vi "Facade.vi"(0 "Data In":T8, 2 "Display State In":T2, 3 "Container State":T7) -> (6 "Data Out":T8, 7 "Display State Out":T2, 8 "Action":T1)   [LabVIEW 2020, in "KTable.xctl"]
uses:
  KTable.xctl
  Data.ctl
  <vilib>/_xctls/Container State.ctl
  State.ctl
  ColumnSpec.ctl
  ColumnType.ctl
  Table Properties.ctl
  Events.ctl
  Event Data.ctl
  Event Type.ctl
  <vilib>/_xctls/Action.ctl
  <vilib>/Utility/miscctls.llb/LVPositionTypeDef.ctl
  <vilib>/_xctls/XControlSupport.lvlib
panel:
  in  "Color":u32(colorbox)
  out "layout":bool
  in  "Ring":u16(ring)
  in  "Listbox":i32(listbox)
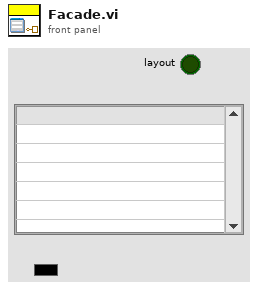
[diagram p1: front panel]
types:
  T1 = typedef "XControlSupport.lvlib/Action.ctl" = cluster{"Data Changed?":bool, "State Changed?":bool, "Action Name":string}
  T2 = typedef "KTable.xctl/State.ctl" = cluster{"Columns":T3[], "Listbox":refnum<vi>, "Default row":string[], "Properties":T5, "Events":T6, "Locked":bool[][], "Size":cluster{"Rows":i32, "Columns":i32}, "rings":i32[][], "DefColors":u32[], "highlight row":bool}
  T3 = typedef "KTable.xctl/ColumnSpec.ctl" = cluster{"Name":string, "Type":T4, "Width":i32, "Strings":string[], "Position":enum16{"Left", "Center", "Right"}, "locked":bool, "cds":cluster{"Strings":string[]}[][], "Hide NaN":bool}
  T4 = typedef "KTable.xctl/ColumnType.ctl" = enum16{"String", "Enum", "Int", "Double", "Boolean", "Ring", "Formula", "Color"}
  T5 = typedef "KTable.xctl/Table Properties.ctl" = cluster{"Vertical scrollbar":bool, "User add/delete":bool, "Max rows":i32, "Row headers":bool}
  T6 = typedef "KTable.xctl/Events.ctl" = cluster{"Items Changed":refnum<user-event>}
  T7 = typedef "XControlSupport.lvlib/Container State.ctl" = cluster{"Indicator?":bool, "Run Mode?":bool, " Refnum":refnum<vi>}
  T8 = typedef "KTable.xctl/Data.ctl" = u16
  T9 = typedef "KTable.xctl/Event Data.ctl" = cluster{"Type":T10, "New row":i32, "Old row":i32, "Data":variant}
  T10 = typedef "KTable.xctl/Event Type.ctl" = enum16{"None", "Selection", "Edit", "Insert", "Delete", "Up", "Down", "Duplicate"}
  T11 = typedef "LVPositionTypeDef.ctl" = cluster{"Left":i32, "Top":i32}
  T12 = typedef "LVRectTypeDef.ctl" = cluster{"Left":i16, "Top":i16, "Right":i16, "Bottom":i16}
  T13 = typedef "LVPoint32TypeDef.ctl" = cluster{"Horizontal":i32, "Vertical":i32}
  T14 = typedef "LVRowAndColumnTypeDef.ctl" = cluster{"Row":i32, "Column":i32}
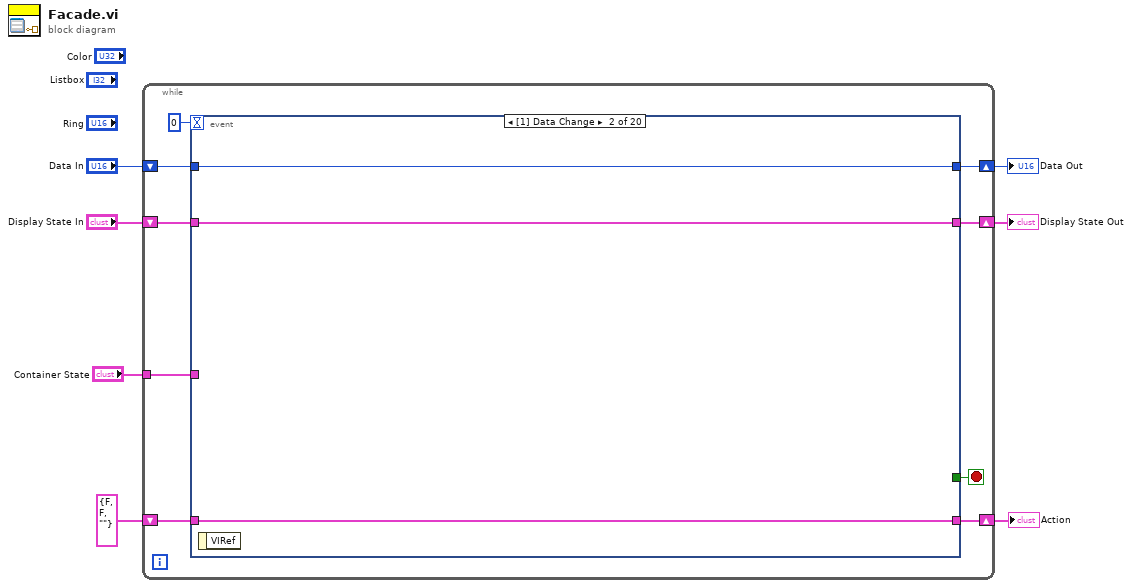
[diagram p0: block diagram]
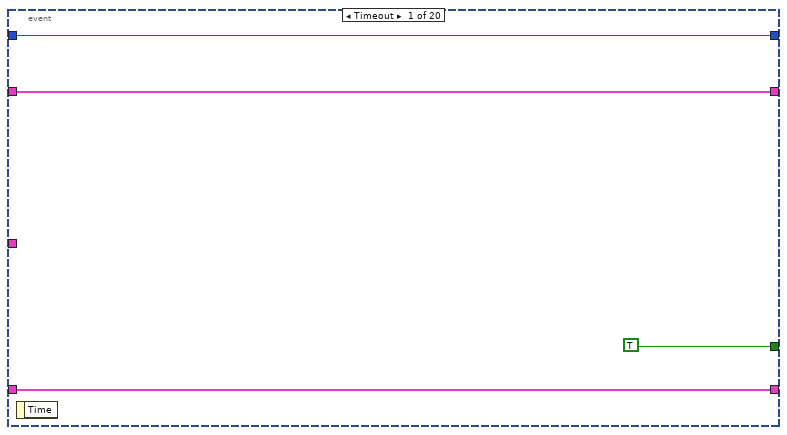
[diagram p2: hidden frame]
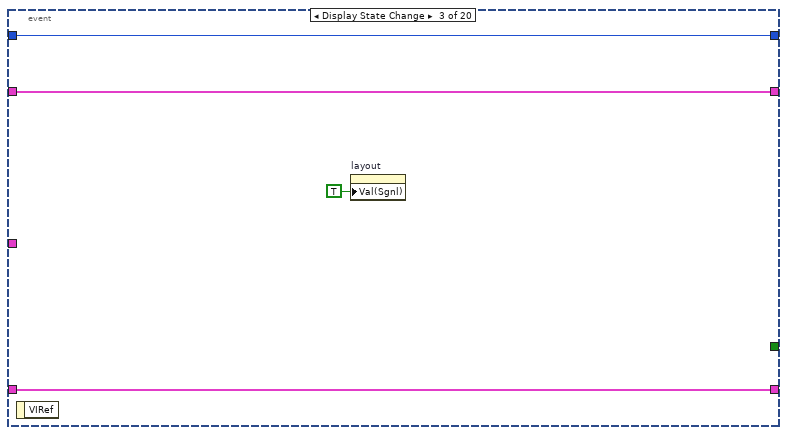
[diagram p3: hidden frame]
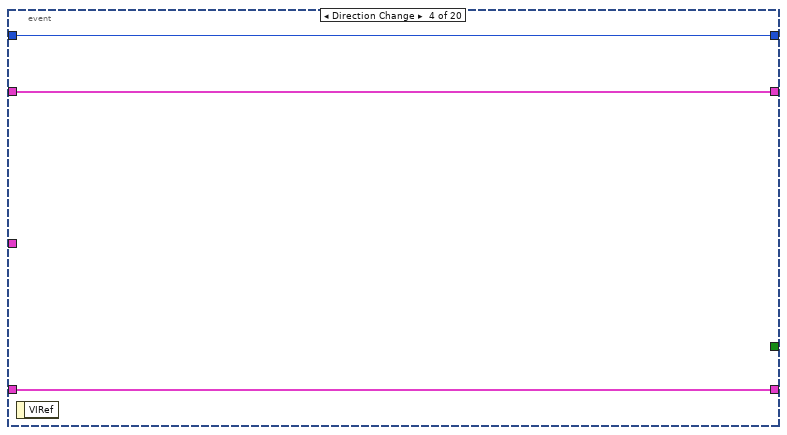
[diagram p4: hidden frame]
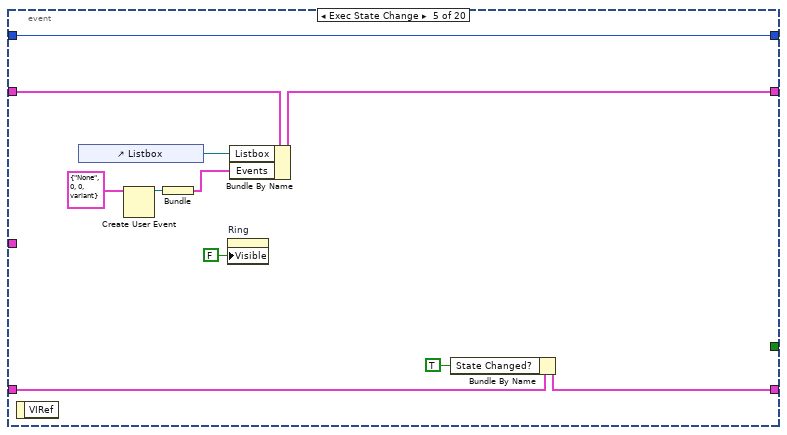
[diagram p5: hidden frame]
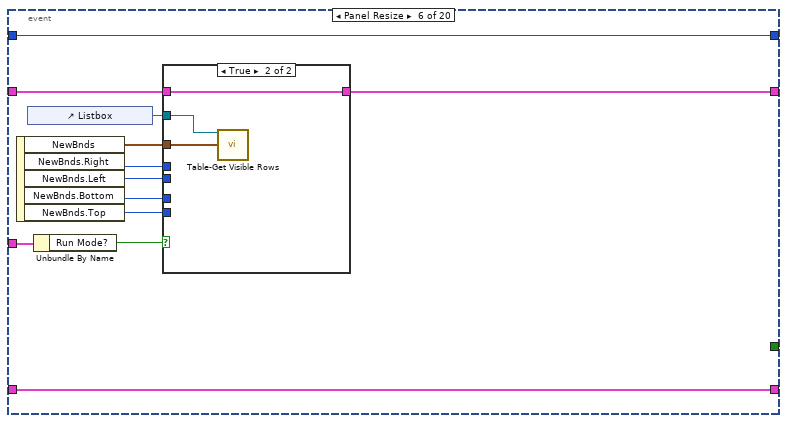
[diagram p6: hidden frame]
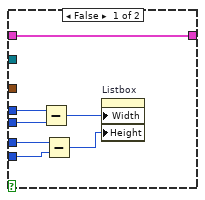
[diagram p7: hidden frame]
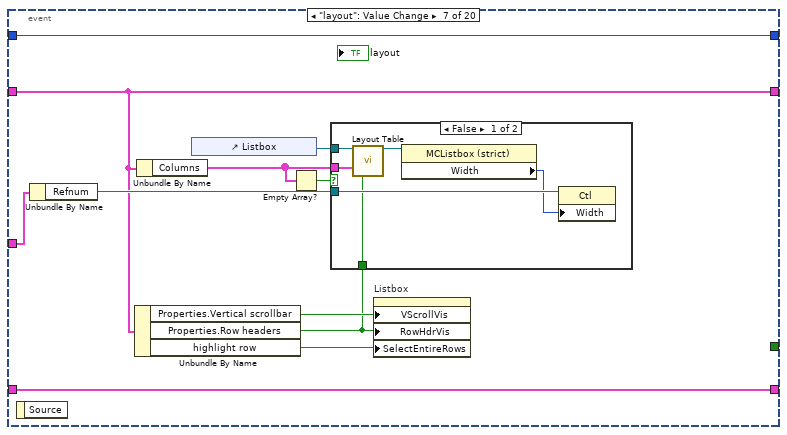
[diagram p8: hidden frame]
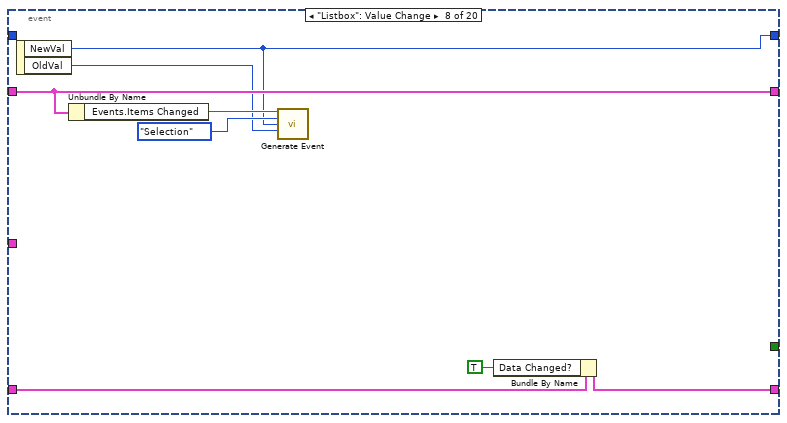
[diagram p10: hidden frame]
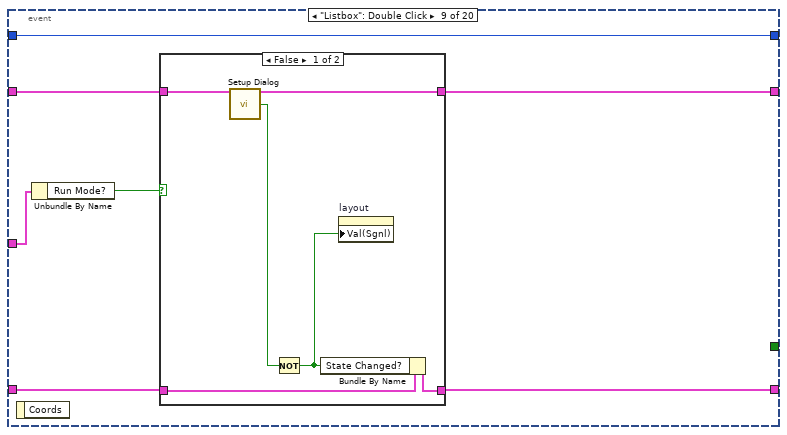
[diagram p11: hidden frame]
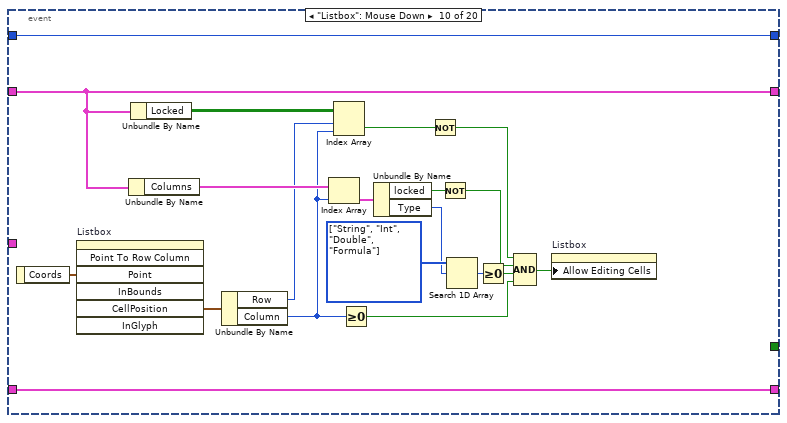
[diagram p13: hidden frame]
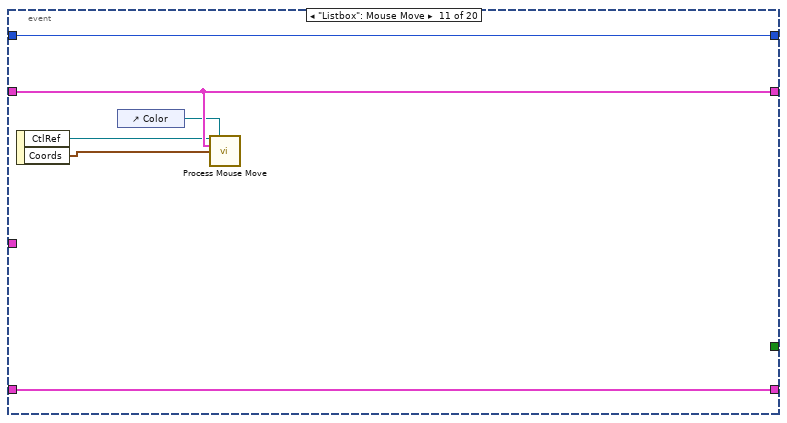
[diagram p14: hidden frame]
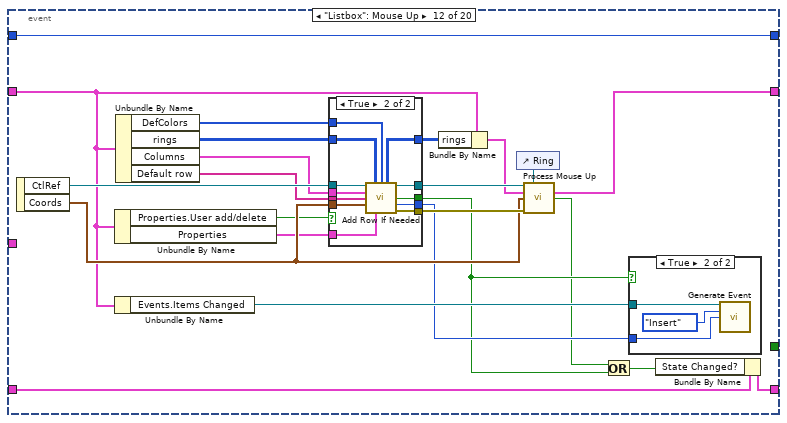
[diagram p15: hidden frame]
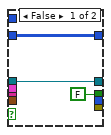
[diagram p16: hidden frame]
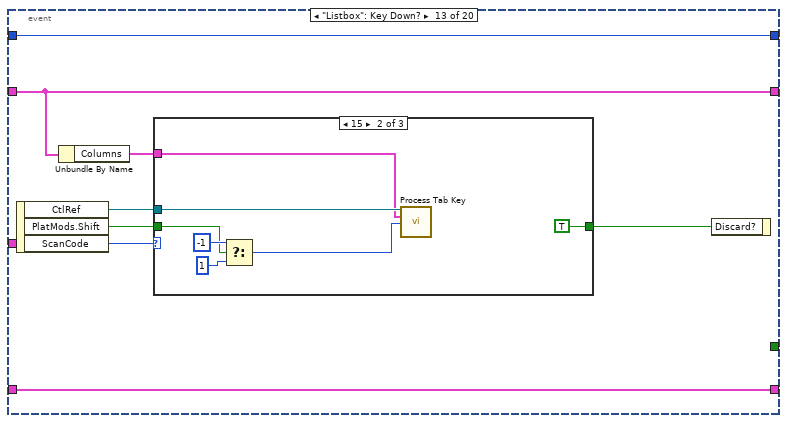
[diagram p18: hidden frame]
diagram:
  n1 = while {
    shift-right: [w15] -> w4
    shift-left: "Display State In" -> [w16]
    tunnel: "Container State" -> [w12]
    shift-right: [w10] -> w7
    shift-left: "Data In" -> [w11]
    shift-right: [w8] -> w2
    shift-left: T1 {"Data Changed?"=FALSE, "State Changed?"=FALSE, "Action Name"=""} ("Action") -> [w9]
    stop <- w14 stop-if-true
    n2 = event shown="[1] Data Change" {
      selector: _ -> [_ _ _ _ _ _ _ _ _ _ _ _ _ _ _ _ _ _ _ _]
      dyn-events: _ -> [_ _ _ _ _ _ _ _ _ _ _ _ _ _ _ _ _ _ _ _]
      timeout: 0 -> [_ _ _ _ _ _ _ _ _ _ _ _ _ _ _ _ _ _ _ _]
      tunnel: w16 -> [w18 w22 w27 w30 w41 w45 w65 w85 w93 w109 w127 w140 w173 w195 w208 w216 w230 w251 w272 w288]
      tunnel: [w18 w22 w27 w30 w38 w44 w65 w85 w89 w109 w127 w131 w173 w195 w208 w216 w230 w245 w272 w288] -> w15
      tunnel: [TRUE _ _ _ _ _ _ _ _ _ _ _ _ _ _ _ _ _ _ _] -> w14
      tunnel: w12 -> [_ _ _ _ _ w47 w71 _ w94 _ _ _ _ _ _ _ _ _ _ _]
      tunnel: w11 -> [w17 w23 w26 w29 w40 w53 w74 _ w95 w123 w129 w152 w178 w202 w212 w218 w236 w264 w284 w287]
      tunnel: [w17 w23 w26 w29 w40 w53 w74 w82 w95 w123 w129 w152 w178 w202 w212 w218 w236 w264 w284 w287] -> w10
      tunnel: [w19 w21 w25 w28 w36 w52 w73 w87 w90 w122 w128 w135 w177 w197 w211 w217 w232 w253 w274 w286] -> w8
      tunnel: w9 -> [w19 w21 w25 w28 w39 w52 w73 w88 w92 w122 w128 w151 w177 w201 w211 w217 w235 w263 w283 w286]
      event Timeout {
        n3 = event-data() -> ()  [unwired: 1 in, 1 out]
      }
      event Data Change {
        n4 = event-data() -> ()  [unwired: 1 in, 1 out]
      }
      event Display State Change {
        n5 = event-data() -> ()  [unwired: 1 in, 1 out]
        n6 = property on="layout" class="Bool (strict)"("Val(Sgnl)"=TRUE ("Value (Signaling)")) -> ()  [unwired: 2 in, 2 out]
      }
      event Direction Change {
        n7 = event-data() -> ()  [unwired: 1 in, 1 out]
      }
      event Exec State Change {
        n8 = event-data() -> ()  [unwired: 1 in, 1 out]
        n9 = control-ref of="Listbox"() -> (w37:refnum<vi>)
        n10 = Create User Event(user event datatype=T9 {"Type"=enum."None", "New row"=0, "Old row"=0, "Data"=variant} ("Event Data")) -> (user event=w33:refnum<user-event>)  [unwired: 1 in, 1 out]
        n11 = Bundle("Event Data"=w33) -> (w31:cluster{"Event Data":refnum<user-event>})  [unwired: 1 in]
        n12 = property on="Ring" class="Ring (strict)"("Visible"=FALSE) -> ()  [unwired: 2 in, 2 out]
        n13 = Bundle By Name(cluster=w41, "Listbox"=w37, "Events"=w31) -> (w38:T2)
        n14 = Bundle By Name(cluster=w39, "State Changed?"=TRUE) -> (w36:T1)
      }
      event Panel Resize {
        n15 = event-data() -> ("NewBnds"=w46:T12, "NewBnds.Right"=w50:i16, "NewBnds.Left"=w51:i16, "NewBnds.Bottom"=w48:i16, "NewBnds.Top"=w49:i16)  [unwired: 1 in]
        n16 = control-ref of="Listbox"() -> (w42:refnum<vi>)
        n17 = Unbundle By Name(w47) -> ("Run Mode?"=w43:bool)
        n18 = case shown="True" w43 {
          tunnel: w51 -> [w60 _]
          tunnel: w50 -> [w59 _]
          tunnel: w49 -> [w58 _]
          tunnel: w48 -> [w57 _]
          tunnel: w46 -> [_ w63]
          tunnel: w45 -> [w54 w61]
          tunnel: [w54 w61] -> w44
          tunnel: w42 -> [_ w62]
          frame False {
            n19 = Subtract(x=w59, y=w60) -> (x-y=w56:i16)
            n20 = Subtract(x=w57, y=w58) -> (x-y=w55:i16)
            n21 = property on="Listbox" class="MCListbox (strict)"("Width"=w56, "Height"=w55) -> ()  [unwired: 2 in, 2 out]
          }
          frame True {
            n22 = call "Table-Get Visible Rows.vi"("reference"=w62, "Bounds"=w63) -> ()  [unwired: 13 in, 1 out]
          }
        }
      }
      event "layout": Value Change {
        n23 = event-data() -> ()  [unwired: 1 in, 1 out]
        n24 = Unbundle By Name(w71) -> ("Refnum"=w70:refnum<vi>)
        n25 = Unbundle By Name(w65) -> ("Properties.Vertical scrollbar"=w67:bool, "Properties.Row headers"=w66:bool, "highlight row"=w64:bool)
        n26 = Unbundle By Name(w65) -> ("Columns"=w69:T3[])
        n27 = control-ref of="Listbox"() -> (w72:refnum<vi>)
        n28 = Empty Array?(array=w69) -> (empty?=w68:bool)
        n29 = case shown="False" w68 {
          tunnel: w72 -> [w80 _]
          tunnel: w70 -> [w78 _]
          tunnel: w69 -> [w76 _]
          tunnel: w66 -> [w75 _]
          frame False {
            n30 = call "Layout Table.vi"("Listbox Ref"=w80, "Columns"=w76, "row headers"=w75) -> ("reference out"=w79:refnum<vi>)  [unwired: 12 in]
            n31 = property class="MCListbox (strict)"(reference=w79) -> ("Width"=w77:u32)  [unwired: 1 in, 2 out]
            n32 = property class="Ctl"(reference=w78, "Width"=w77) -> ()  [unwired: 1 in, 2 out]
          }
          frame True {
          }
        }
        n33 = property on="Listbox" class="MCListbox (strict)"("VScrollVis"=w67, "RowHdrVis"=w66, "SelectEntireRows"=w64) -> ()  [unwired: 2 in, 2 out]
      }
      event "Listbox": Value Change {
        n34 = event-data() -> ("NewVal"=w82:i32, "OldVal"=w81:i32)  [unwired: 1 in]
        n35 = Unbundle By Name(w85) -> ("Events.Items Changed"=w84:refnum<user-event>)
        n36 = call "Generate Event.vi"("Event"=w84, "Type"=Event_Type."Selection", "New row"=w82, "Old row"=w81) -> ()  [unwired: 11 in, 1 out]
        n37 = Bundle By Name(cluster=w88, "Data Changed?"=TRUE) -> (w87:T1)
      }
      event "Listbox": Double Click {
        n38 = event-data() -> ()  [unwired: 1 in, 1 out]
        n39 = Unbundle By Name(w94) -> ("Run Mode?"=w91:bool)
        n40 = case shown="False" w91 {
          tunnel: w93 -> [w101 w102]
          tunnel: w92 -> [w99 w103]
          tunnel: [w98 w103] -> w90
          tunnel: [w100 w102] -> w89
          frame False {
            n41 = call "Setup Dialog.vi"("State In"=w101) -> ("State Out"=w100:T2, "canceled?"=w97:bool)  [unwired: 13 in]
            n42 = Not(x=w97) -> (.not. x?=w96:bool)
            n43 = Bundle By Name(cluster=w99, "State Changed?"=w96) -> (w98:T1)
            n44 = property on="layout" class="Bool (strict)"("Val(Sgnl)"=w96) -> ()  [unwired: 2 in, 2 out]
          }
          frame True {
          }
        }
      }
      event "Listbox": Mouse Down {
        w117 = T4[] [enum."String", enum."Int", enum."Double", enum."Formula"] items=["String", "Enum", "Int", "Double", "Boolean", "Ring", "Formula", "Color"] ("y")
        n45 = event-data() -> ("Coords"=w121:T13)  [unwired: 1 in]
        n46 = invoke on="Listbox" class="MCListbox (strict)" method="Point To Row Column"("Point"=w121) -> ("CellPosition"=w119:T14)  [unwired: 6 in, 6 out]
        n47 = Unbundle By Name(w109) -> ("Columns"=w120:T3[])
        n48 = Unbundle By Name(w109) -> ("Locked"=w113:bool[][])
        n49 = Unbundle By Name(w119) -> ("Row"=w112:i32, "Column"=w105:i32)
        n50 = Index Array(array=w120, index=w105) -> (element=w118:T3)
        n51 = Index Array(array=w113, index (row)=w112, index (col)=w105) -> (element=w110:bool)
        n52 = Greater Or Equal To 0?(x=w105) -> (x >= 0?=w104:bool)
        n53 = Unbundle By Name(w118) -> ("locked"=w107:bool, "Type"=w116:T4)
        n54 = Not(x=w110) -> (.not. x?=w108:bool)
        n55 = Not(x=w107) -> (.not. x?=w106:bool)
        n56 = Search 1D Array(1D array=w117, element=w116) -> (index of element=w115:i32)  [unwired: 1 in]
        n57 = Greater Or Equal To 0?(x=w115) -> (x >= 0?=w114:bool)
        n58 = Compound Arithmetic op=AND(w108, w106, w114, w104) -> (w111:bool)
        n59 = property on="Listbox" class="MCListbox (strict)"("Allow Editing Cells"=w111) -> ()  [unwired: 2 in, 2 out]
      }
      event "Listbox": Mouse Move {
        n60 = event-data() -> ("CtlRef"=w125:refnum<vi>, "Coords"=w124:T13)  [unwired: 1 in]
        n61 = control-ref of="Color"() -> (w126:refnum<vi>)
        n62 = call "Process Mouse Move.vi"("Listbox"=w125, "Color Box"=w126, "State in"=w127, "Coords"=w124) -> ()  [unwired: 10 in, 2 out]
      }
      event "Listbox": Mouse Up {
        n63 = event-data() -> ("CtlRef"=w149:refnum<vi>, "Coords"=w145:T13)  [unwired: 1 in]
        n64 = Unbundle By Name(w140) -> ("Properties.User add/delete"=w142:bool, "Properties"=w139:T5)
        n65 = Unbundle By Name(w140) -> ("Events.Items Changed"=w144:refnum<user-event>)
        n66 = Unbundle By Name(w140) -> ("DefColors"=w130:u32[], "rings"=w138:i32[][], "Columns"=w141:T3[], "Default row"=w147:string[])
        n67 = case shown="True" w142 {
          tunnel: w149 -> [w155 w167]
          tunnel: [w155 w166] -> w148
          tunnel: w147 -> [_ w165]
          tunnel: [_ w164] -> w146
          tunnel: w145 -> [_ w163]
          tunnel: w141 -> [_ w162]
          tunnel: [FALSE ("row added?") w161] -> w133
          tunnel: [_ w160] -> w143
          tunnel: w139 -> [_ w159]
          tunnel: w138 -> [w153 w158]
          tunnel: [w153 w157] -> w136
          tunnel: w130 -> [_ w156]
          frame False {
          }
          frame True {
            n68 = call "Add Row If Needed.vi"("Listbox In"=w167, "rings in"=w158, "DefColors"=w156, "Columns"=w162, "Default"=w165, "Coords"=w163, "Properties"=w159) -> ("rings out"=w157:i32[][], "Listbox out"=w166:refnum<vi>, "row added?"=w161:bool, "Row"=w160:i32, "error out"=w164:errorcluster)  [unwired: 4 in]
          }
        }
        n69 = Bundle By Name(cluster=w140, "rings"=w136) -> (w137:T2)
        n70 = control-ref of="Ring"() -> (w150:refnum<vi>)
        n71 = call "Process Mouse Up.vi"("Listbox"=w148, "Ring"=w150, "State in"=w137, "Coords"=w145, "error in (no error)"=w146) -> ("State out"=w131:T2, "state changed"=w132:bool)  [unwired: 8 in, 1 out]
        n72 = Or(x=w132, y=w133) -> (x .or. y?=w134:bool)
        n73 = case shown="True" w133 {
          tunnel: w144 -> [_ w170]
          tunnel: w143 -> [_ w168]
          frame False {
          }
          frame True {
            n74 = call "Generate Event.vi"("Event"=w170, "Type"=Event_Type."Insert", "New row"=w168) -> ()  [unwired: 12 in, 1 out]
          }
        }
        n75 = Bundle By Name(cluster=w151, "State Changed?"=w134) -> (w135:T1)
      }
      event "Listbox": Key Down? {
        n76 = event-data() -> ("CtlRef"=w171:refnum<vi>, "PlatMods.Shift"=w174:bool, "ScanCode"=w176:i16)  [unwired: 1 in]
        n77 = Unbundle By Name(w173) -> ("Columns"=w172:T3[])
        n78 = case shown="15" w176 {
          tunnel: [_ TRUE ("Shift") w186] -> w175
          tunnel: w174 -> [_ w183 w186]
          tunnel: w172 -> [_ w180 _]
          tunnel: w171 -> [_ w181 _]
          frame 0, Default {
          }
          frame 15 {
            n79 = Select(t=-1, s=w183, f=1) -> (s? t:f=w179:i32)
            n80 = call "Process Tab Key.vi"("MulticolumnListbox in"=w181, "Columns"=w180, "increment"=w179) -> ()  [unwired: 13 in]
          }
          frame 72, 80 {
          }
        }
        n81 = event-data("Discard?"=w175) -> ()  [unwired: 1 in, 1 out]
      }
      event "Listbox": Key Up {
        n82 = event-data() -> ("PlatMods.Shift"=w194:bool, "CtlRef"=w199:refnum<vi>, "ScanCode"=w200:i16)  [unwired: 1 in]
        n83 = local read "Listbox"() -> (w198:i32)
        n84 = Unbundle By Name(w195) -> ("Properties.User add/delete"=w193:bool)
        n85 = And(x=w193, y=w194) -> (x .and. y?=w187:bool)
        n86 = Unbundle By Name(w195) -> ("Events.Items Changed"=w192:refnum<user-event>)
        n87 = Unbundle By Name(w195) -> ("Properties"=w189:T5, "Columns"=w188:T3[])
        n88 = call "Process Keystroke.vi"("Listbox"=w199, "can move"=w187, "ScanCode"=w200, "Row"=w198, "Properties"=w189, "Columns"=w188) -> ("Event type"=w191:T10, "Row Out"=w190:i32, "data changed?"=w196:bool)  [unwired: 6 in, 1 out]
        n89 = case shown="True" w196 {
          tunnel: w192 -> [_ w206]
          tunnel: w191 -> [_ w205]
          tunnel: w190 -> [_ w204]
          tunnel: w198 -> [_ w203]
          frame False {
          }
          frame True {
            n90 = call "Generate Event.vi"("Event"=w206, "Type"=w205, "New row"=w204, "Old row"=w203) -> ()  [unwired: 11 in, 1 out]
          }
        }
        n91 = Bundle By Name(cluster=w201, "Data Changed?"=w196) -> (w197:T1)
      }
      event "Listbox": Edit Cell {
        n92 = event-data() -> ("Coords.Row"=w207:i32)  [unwired: 1 in]
        n93 = Unbundle By Name(w208) -> ("Events.Items Changed"=w210:refnum<user-event>)
        n94 = call "Generate Event.vi"("Event"=w210, "Type"=Event_Type."Edit", "New row"=w207) -> ()  [unwired: 12 in, 1 out]
      }
      event "Listbox": Shortcut Menu Activation? {
        n95 = event-data() -> ("MenuRef"=w215:refnum<k9>)  [unwired: 1 in]
        n96 = Unbundle By Name(w216) -> ("Properties.User add/delete"=w213:bool)
        n97 = Not(x=w213) -> (.not. x?=w214:bool)
        n98 = case shown="True" w213 {
          tunnel: w215 -> [_ w223]
          frame False {
          }
          frame True {
            n99 = Delete Menu Items(9:w223) -> (0:w222:errorcluster, 3:w221:refnum<k9>)  [unwired: 3 in]
            n100 = Insert Menu Items(6:w222, 7:string[] ["sc_delete_row", "sc_delete_all", "sc_duplicate_row"] ("item tags"), 8:string[] ["Delete selected row", "Delete all rows", "Duplicate selected row"] ("item names"), 9:w221) -> ()  [unwired: 2 in, 3 out]
          }
        }
        n101 = event-data("Discard?"=w214) -> ()  [unwired: 1 in, 1 out]
      }
      event "Listbox": Shortcut Menu Selection (User) {
        n102 = event-data() -> ("CtlRef"=w234:refnum<vi>, "ItemTag"=w225:string)  [unwired: 1 in]
        n103 = local read "Listbox"() -> (w233:i32)
        n104 = Unbundle By Name(w230) -> ("Events.Items Changed"=w229:refnum<user-event>)
        n105 = Unbundle By Name(w230) -> ("Properties"=w226:T5, "Columns"=w224:T3[])
        n106 = call "Process Menu.vi"("Listbox"=w234, "menu tag"=w225, "Row"=w233, "Properties"=w226, "Columns"=w224) -> ("Event type"=w228:T10, "Row Out"=w227:i32, "data changed?"=w231:bool)  [unwired: 7 in, 1 out]
        n107 = case shown="True" w231 {
          tunnel: w229 -> [_ w240]
          tunnel: w228 -> [_ w239]
          tunnel: w227 -> [_ w238]
          tunnel: w233 -> [_ w237]
          frame False {
          }
          frame True {
            n108 = call "Generate Event.vi"("Event"=w240, "Type"=w239, "New row"=w238, "Old row"=w237) -> ()  [unwired: 11 in, 1 out]
          }
        }
        n109 = Bundle By Name(cluster=w235, "Data Changed?"=w231) -> (w232:T1)
      }
      event "Ring": Value Change {
        n110 = event-data() -> ("CtlRef"=w259:refnum<vi>)  [unwired: 1 in]
        n111 = Unbundle By Name(w251) -> ("Events.Items Changed"=w255:refnum<user-event>)
        n112 = property on="Property Node" class="Ring (strict)"(reference=w259, "Visible"=FALSE) -> ("Position"=w261:T11, "RingText.Text"=w256:string, "Value"=w248:u16)  [unwired: 1 in, 2 out]
        n113 = Add(x=T11 {"Left"=10, "Top"=10} ("y"), y=w261) -> (x+y=w262:T11)
        n114 = call "Generate Event.vi"("Event"=w255, "Type"=Event_Type."Edit") -> ()  [unwired: 13 in, 1 out]
        n115 = invoke on="Listbox" class="MCListbox (strict)" method="Point To Row Column"("Point"=w262) -> ("CellPosition"=w242:T14)  [unwired: 6 in, 6 out]
        n116 = property on="Listbox" class="MCListbox (strict)"() -> ("ItemNames"=w257:string[][])  [unwired: 2 in, 2 out]
        n117 = Unbundle(w242) -> ("Row"=w249:i32, "Column"=w241:i32)
        n118 = Unbundle By Name(w251) -> ("rings"=w250:i32[][])
        n119 = Replace Array Subset(array=w257, new element=w256, index (row)=w249, index (col)=w241) -> (w244:string[][])
        n120 = Bundle By Name(cluster=w263, "State Changed?"=TRUE) -> (w253:T1)
        n121 = Replace Array Subset(array=w250, new element=w248, index (row)=w249, index (col)=w241) -> (w247:i32[][])
        n122 = Bundle By Name(cluster=w251, "rings"=w247) -> (w246:T2)
        n123 = call "Check Context Dependent Rings.vi"("Display State in"=w246, "ItemNames in"=w244, "CellPosition"=w242) -> ("Display State out"=w245:T2, "ItemNames out"=w243:string[][])  [unwired: 11 in]
        n124 = property on="Listbox" class="MCListbox (strict)"("ItemNames"=w243) -> ()  [unwired: 2 in, 2 out]
      }
      event "Color": Value Change {
        n125 = event-data() -> ("CtlRef"=w279:refnum<vi>)  [unwired: 1 in, 2 out]
        n126 = Unbundle By Name(w272) -> ("Events.Items Changed"=w276:refnum<user-event>)
        n127 = property on="Property Node" class="ColBox"(reference=w279, "Visible"=FALSE) -> ("Position"=w281:T11, "Value"=w265:u32)  [unwired: 1 in, 2 out]
        n128 = Add(x=T11 {"Left"=10, "Top"=10} ("y"), y=w281) -> (x+y=w282:T11)
        n129 = call "Generate Event.vi"("Event"=w276, "Type"=Event_Type."Edit") -> ()  [unwired: 13 in, 1 out]
        n130 = invoke on="Listbox" class="MCListbox (strict)" method="Point To Row Column"("Point"=w282) -> ("CellPosition"=w266:T14)  [unwired: 6 in, 6 out]
        n131 = property on="Listbox" class="MCListbox (strict)"() -> ("ItemNames"=w277:string[][])  [unwired: 2 in, 2 out]
        n132 = Format Into String(format string="%06x", w265) -> (resulting string=w268:string)  [unwired: 2 in, 1 out]
        n133 = Unbundle(w266) -> ("Row"=w271:i32, "Column"=w269:i32)
        n134 = Replace Array Subset(array=w277, new element=w268, index (row)=w271, index (col)=w269) -> (w270:string[][])
        n135 = Bundle By Name(cluster=w283, "State Changed?"=TRUE) -> (w274:T1)
        n136 = property on="Listbox" class="MCListbox (strict)"("ItemNames"=w270, "ActiveCell"=w266, "CellBG"=w265) -> ()  [unwired: 2 in, 2 out]
      }
      event Mouse Leave {
        n137 = event-data() -> ()  [unwired: 1 in, 1 out]
        n138 = property on="Ring" class="Ring (strict)"("Visible"=FALSE) -> ()  [unwired: 2 in, 2 out]
      }
    }
  }
  "Display State Out" <- w4
  "Data Out" <- w7
  "Action" <- w2
